vi "WSVCAP SHL Host LL I2C Convert 4 Bytes to Status and Capacitance.vi"(0 "C1:1-16 Read Data [U8]":u8[][](array[numeric]) format="%.0x", 5 "C2_1-16 Read Data [U8]":u8[][](array[numeric]) format="%.0x", 7 "C3_1-16 Read Data [U8]":u8[][](array[numeric]) format="%.0x") -> (4 "AD7747 Values":string[][](table))   [LabVIEW 2012]
panel:
  out "Data Headers":u8[](array[numeric])=[1, 2, 3, 4, 5, 6, 7, 8, 9, 10, 11, 12, 12, 14, 15, 16]
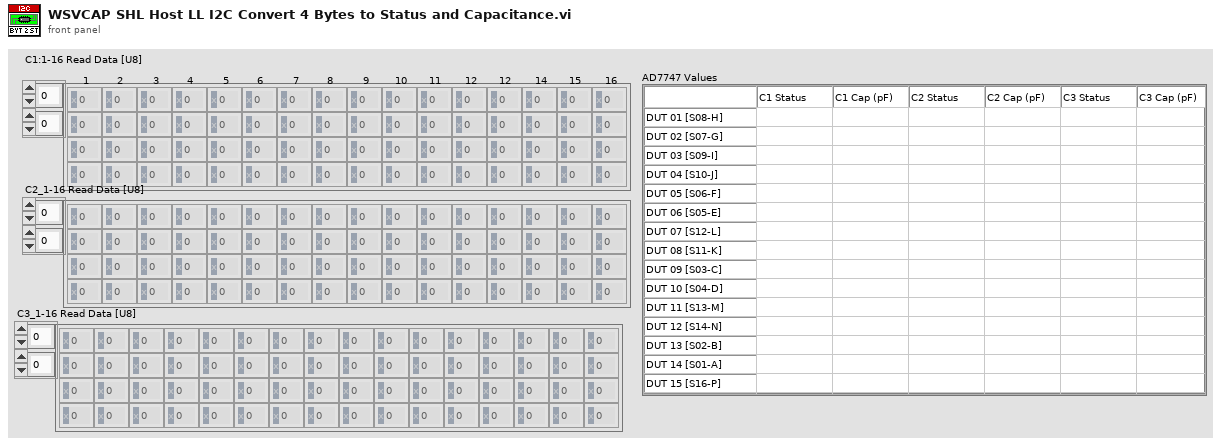
[diagram p1: front panel]
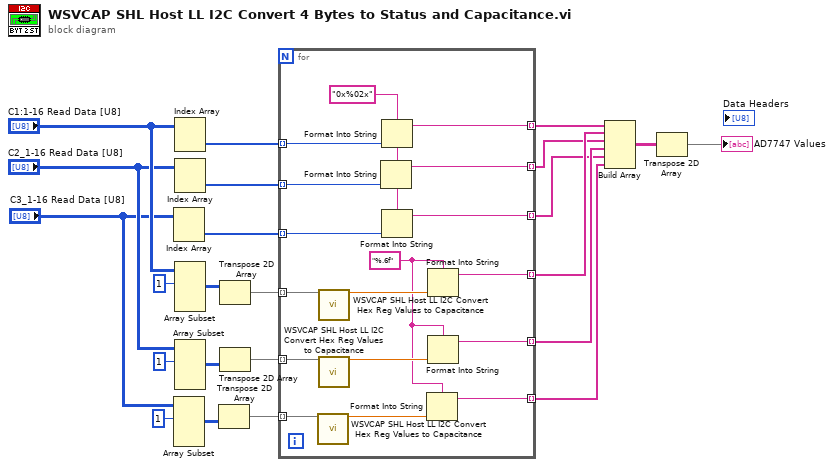
[diagram p0: block diagram]
diagram:
  n1 = Index Array(array="C3_1-16 Read Data [U8]") -> (element=w3:u8[])  [unwired: 2 in]
  n2 = Array Subset(array="C3_1-16 Read Data [U8]", index (row)=1 ("index")) -> (w6:u8[][])  [unwired: 3 in]
  n3 = Index Array(array="C1:1-16 Read Data [U8]") -> (element=w22:u8[])  [unwired: 2 in]
  n4 = Index Array(array="C2_1-16 Read Data [U8]") -> (element=w23:u8[])  [unwired: 2 in]
  n5 = Array Subset(array="C1:1-16 Read Data [U8]", index (row)=1 ("index")) -> (w17:u8[][])  [unwired: 3 in]
  n6 = Array Subset(array="C2_1-16 Read Data [U8]", index (row)=1 ("index")) -> (w16:u8[][])  [unwired: 3 in]
  n7 = Transpose 2D Array(2D array=w6) -> (transposed array=w7:u8[][])
  n8 = Transpose 2D Array(2D array=w17) -> (transposed array=w15:u8[][])
  n9 = Transpose 2D Array(2D array=w16) -> (transposed array=w14:u8[][])
  n10 = for {
    tunnel: w23 -> [w37] mode=indexing
    tunnel: w22 -> [w38] mode=indexing
    tunnel: w15 -> [w40] mode=indexing
    tunnel: w14 -> [w39] mode=indexing
    tunnel: [w34] -> w13 mode=indexing
    tunnel: [w33] -> w12 mode=indexing
    tunnel: [w32] -> w11 mode=indexing
    tunnel: [w31] -> w10 mode=indexing
    tunnel: w7 -> [w27] mode=indexing
    tunnel: [w29] -> w1 mode=indexing
    tunnel: w3 -> [w26] mode=indexing
    tunnel: [w25] -> w2 mode=indexing
    w24 = "%.6f" ("format string")
    w30 = "0x%02x" ("format string")
    n11 = call "WSVCAP SHL Host LL I2C Convert Hex Reg Values to Capacitance.vi"("Bytes (H-M-L)"=w27) -> ("Capacitance (pF)"=w28:dbl)  [unwired: 14 in]
    n12 = call "WSVCAP SHL Host LL I2C Convert Hex Reg Values to Capacitance.vi"("Bytes (H-M-L)"=w40) -> ("Capacitance (pF)"=w36:dbl)  [unwired: 14 in]
    n13 = call "WSVCAP SHL Host LL I2C Convert Hex Reg Values to Capacitance.vi"("Bytes (H-M-L)"=w39) -> ("Capacitance (pF)"=w35:dbl)  [unwired: 14 in]
    n14 = Format Into String(format string=w30, w37) -> (resulting string=w32:string)  [unwired: 2 in, 1 out]
    n15 = Format Into String(format string=w30, w38) -> (resulting string=w34:string)  [unwired: 2 in, 1 out]
    n16 = Format Into String(format string=w30, w26) -> (resulting string=w25:string)  [unwired: 2 in, 1 out]
    n17 = Format Into String(format string=w24, w28) -> (resulting string=w29:string)  [unwired: 2 in, 1 out]
    n18 = Format Into String(format string=w24, w36) -> (resulting string=w33:string)  [unwired: 2 in, 1 out]
    n19 = Format Into String(format string=w24, w35) -> (resulting string=w31:string)  [unwired: 2 in, 1 out]
  }
  n20 = Build Array(w13, w12, w11, w10, w2, w1) -> (w9:string[][])
  n21 = Transpose 2D Array(2D array=w9) -> (transposed array=→"AD7747 Values":string[][])
